vi "GV-StartPreset.vi"(8 "error in (no error)":errorcluster, 11 "Gviewer in":refnum<class "Gviewer.lvclass">) -> (0 "error out":errorcluster, 3 "Gviewer out":refnum<class "Gviewer.lvclass">)   [LabVIEW 2020, in "Sgraph_lib_V1.lvlib" / "Gviewer.lvclass"]
uses:
  Gviewer.lvclass
  Gviewer.lvclass/Gviewer.ctl
  controls/EditTagOneTag.ctl
panel:
  in  "Selector":i32[](listbox)
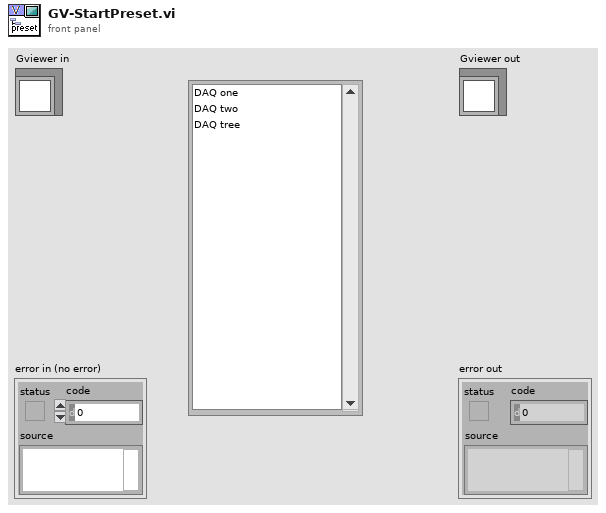
[diagram p1: front panel]
types:
  T1 = cluster{"Editor_ref":refnum<vi>, "Cnt_names":string[], "Cnt_refs":refnum<vi>[]}
  T2 = enum32{"Invalid", "Standard", "Closed", "Hidden", "Minimized", "Maximized"}
  T3 = typedef "Sgraph_lib_V1.lvlib/Gviewer.lvclass/EditTagOneTag.ctl" = cluster{"TAG":string, "min":dbl, "max":dbl, "Color":u32}
  T4 = typedef "Sgraph_lib_V1.lvlib/Gviewer.lvclass/Typedef_SelProperties.ctl" = cluster{"Color":u32, "LineType":T5, "max":dbl, "min":dbl}
  T5 = typedef "Sgraph_lib_V1.lvlib/Gviewer.lvclass/Typedef_LineType.ctl" = enum16{"num_bare", "num_MinMax_Area", "num_MinMax_Lines", "num_MinMax_Forfor", "num_Max_Area", "num_Max_Line", "num_Max_Forfor", "num_Min_Area", "num_Min_Line", "num_Min_Fosfor", "Boolean_Line_01", "Boolean_Area_01", "Boolean_Fosfor_01", "Boolean_Line_TF", "Boolean_Area_TF", "Boolean_Fosfor_TF", "Boolean_OnOff_Line", "Boolean_OnOff_Area", "Boolean_OnOff_Fosfor", "Boolean_spare", "StringEvent_Line", "StringEvent_TimeLine"}
  T6 = typedef "Sgraph_lib_V1.lvlib/DBAL_TAGprops.ctl" = T7[]
  T7 = typedef "Sgraph_lib_V1.lvlib/DBAL_TAGpropEdit.ctl" = cluster{"TAG":string, "Qtype":string, "TAGprop":T8}
  T8 = typedef "Sgraph_lib_V1.lvlib/typedef_com_TagProp.ctl" = cluster{"Description":string, "EngUnits":string, "RangeH":dbl, "RangeL":dbl, "Resolution":i32, "Obsolete":bool, "ChangeDate":timestamp, "ChangeSource":string, "ChangeReason":string, "TagFunc":u32}
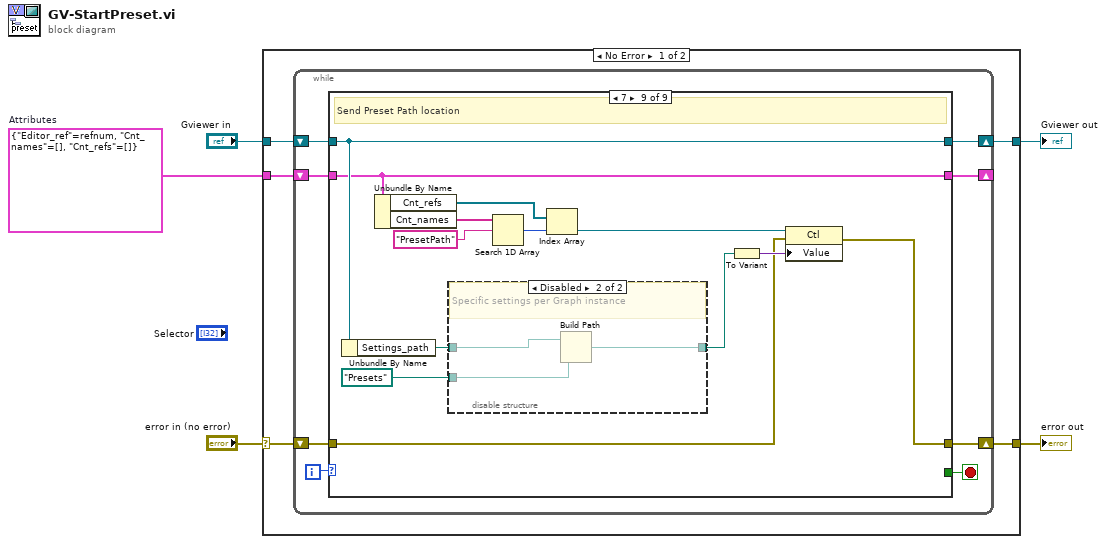
[diagram p0: block diagram]
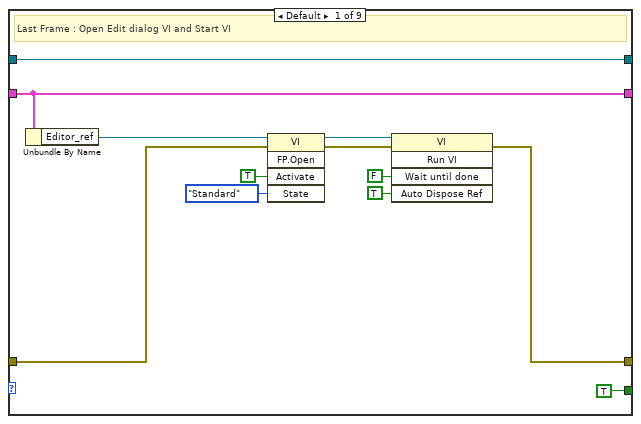
[diagram p2: hidden frame]
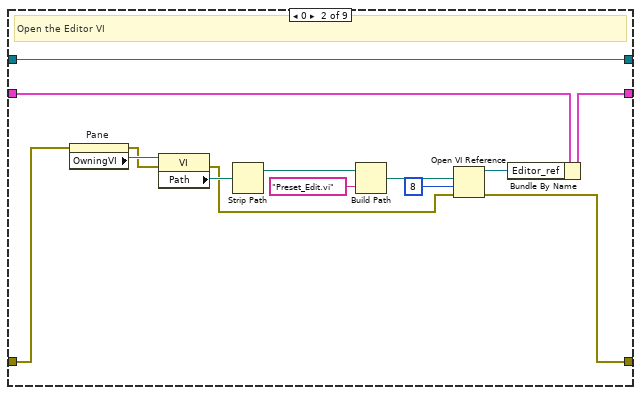
[diagram p3: hidden frame]
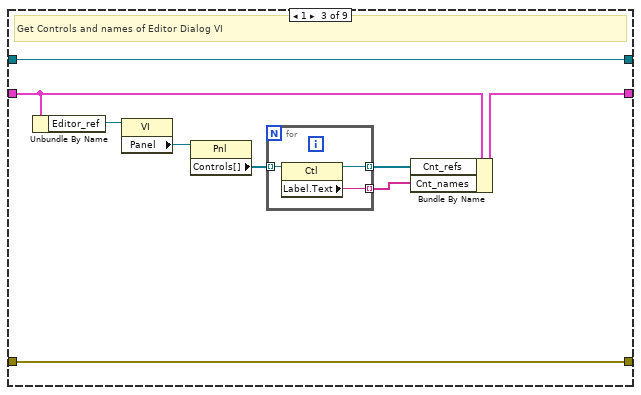
[diagram p4: hidden frame]
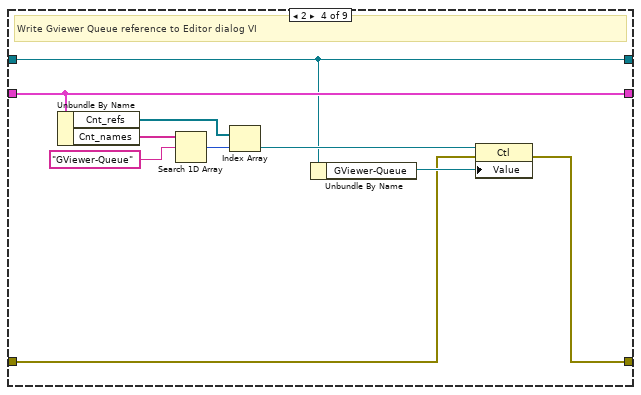
[diagram p5: hidden frame]
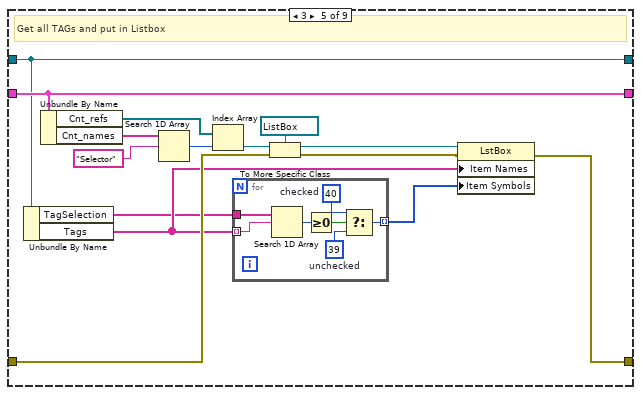
[diagram p6: hidden frame]
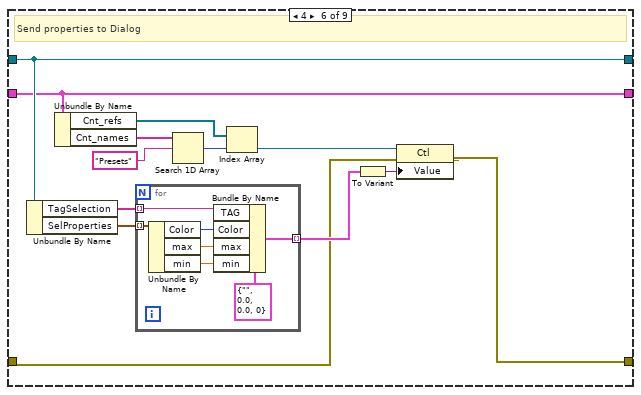
[diagram p7: hidden frame]
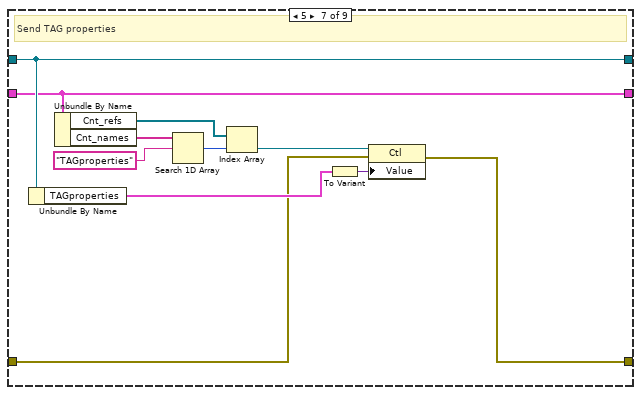
[diagram p8: hidden frame]
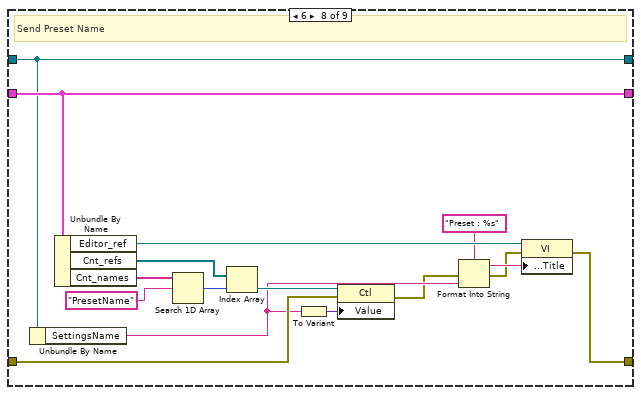
[diagram p9: hidden frame]
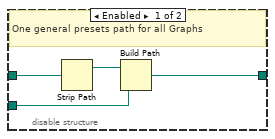
[diagram p10: hidden frame]
diagram:
  w1 = T1 {"Editor_ref"=refnum, "Cnt_names"=[], "Cnt_refs"=[]}  # Attributes
  n1 = case shown="No Error" "error in (no error)" {
    selector: "error in (no error)" -> [w9 w157]
    tunnel: [w7 w157] -> w4
    tunnel: [w8 w156] -> w2
    tunnel: "Gviewer in" -> [w10 w156]
    tunnel: w1 -> [w6 _]
    frame No Error {
      n2 = while {
        shift-right: [w15] -> w8
        shift-left: w10 -> [w17]
        shift-right: [w14] -> w7
        shift-left: w9 -> [w16]
        shift-right: [w11] -> _
        shift-left: w6 -> [w12]
        i -> [w18]
        stop <- w13 stop-if-true
        n3 = case shown="7" w18 {
          tunnel: w17 -> [w30 w44 w53 w59 w73 w101 w119 w125 w148]
          tunnel: w16 -> [w26 w31 w52 w57 w70 w89 w109 w128 w139]
          tunnel: [w30 w44 w53 w59 w73 w101 w119 w125 w148] -> w15
          tunnel: [w21 w35 w52 w58 w71 w91 w112 w126 w141] -> w14
          tunnel: [TRUE _ _ _ _ _ _ _ _] -> w13
          tunnel: [w28 w38 w46 w61 w74 w94 w114 w131 w143] -> w11
          tunnel: w12 -> [w28 w39 w45 w61 w74 w94 w114 w131 w143]
          frame Default {
            # "Last Frame : Open Edit dialog VI and Start VI"
            n4 = Unbundle By Name(w28) -> ("Editor_ref"=w25:refnum<vi>)
            n5 = invoke class="VI" method="FP.Open"(reference=w25, error in=w26, "Activate"=TRUE ("Wait Until Done"), "State"=T2."Standard") -> (reference out=w23:refnum<vi>, error out=w22:errorcluster)  [unwired: 1 in, 3 out]
            n6 = invoke class="VI" method="Run VI"(reference=w23, error in=w22, "Wait until done"=FALSE ("Wait Until Done"), "Auto Dispose Ref"=TRUE ("Auto Dispose Reference")) -> (error out=w21:errorcluster)  [unwired: 1 in, 4 out]
          }
          frame 0 {
            # "Open the Editor VI"
            n7 = property on="Pane" class="Pane"(error in=w31) -> (error out=w32:errorcluster, "OwningVI"=w33:refnum<vi>)  [unwired: 1 in, 1 out]
            n8 = property class="VI"(reference=w33, error in=w32) -> (error out=w36:errorcluster, "Path"=w43:path)  [unwired: 1 out]
            n9 = Strip Path(path=w43) -> (stripped path=w42:path)  [unwired: 1 out]
            n10 = Build Path(base path=w42, name or relative path="Preset_Edit.vi") -> (appended path=w40:path)
            n11 = Open VI Reference(vi path=w40, options=8, error in (no error)=w36) -> (vi reference=w37:refnum<vi>, error out=w35:errorcluster)  [unwired: 3 in]
            n12 = Bundle By Name(cluster=w39, "Editor_ref"=w37) -> (w38:T1)
          }
          frame 1 {
            # "Get Controls and names of Editor Dialog VI"
            n13 = Unbundle By Name(w45) -> ("Editor_ref"=w51:refnum<vi>)
            n14 = property class="VI"(reference=w51) -> ("Panel"=w50:refnum<vi>)  [unwired: 1 in, 2 out]
            n15 = property class="Pnl"(reference=w50) -> ("Controls[]"=w49:refnum<vi>[])  [unwired: 1 in, 2 out]
            n16 = for {
              tunnel: w49 -> [w56] mode=indexing
              tunnel: [w55] -> w47 mode=indexing
              tunnel: [w54] -> w48 mode=indexing
              n17 = property class="Ctl"(reference=w56) -> (reference out=w55:refnum<vi>, "Label.Text"=w54:string)  [unwired: 1 in, 1 out]
            }
            n18 = Bundle By Name(cluster=w45, "Cnt_refs"=w47, "Cnt_names"=w48) -> (w46:T1)
          }
          frame 2 {
            # "Write Gviewer Queue reference to Editor dialog VI"
            n19 = Unbundle By Name(w61) -> ("Cnt_refs"=w64:refnum<vi>[], "Cnt_names"=w66:string[])
            n20 = Search 1D Array(1D array=w66, element="GViewer-Queue") -> (index of element=w63:i32)  [unwired: 1 in]
            n21 = Index Array(array=w64, index=w63) -> (element=w62:refnum<vi>)
            n22 = Unbundle By Name(w59) -> ("GViewer-Queue"=w60:refnum<queue>)
            n23 = property class="Ctl"(reference=w62, error in=w57, "Value"=w60) -> (error out=w58:errorcluster)  [unwired: 1 out]
          }
          frame 3 {
            # "Get all TAGs and put in Listbox"
            n24 = Unbundle By Name(w73) -> ("TagSelection"=w68:string[], "Tags"=w69:string[])
            n25 = Unbundle By Name(w74) -> ("Cnt_refs"=w80:refnum<vi>[], "Cnt_names"=w81:string[])
            n26 = Search 1D Array(1D array=w81, element="Selector") -> (index of element=w79:i32)  [unwired: 1 in]
            n27 = Index Array(array=w80, index=w79) -> (element=w77:refnum<vi>)
            n28 = for {
              tunnel: w69 -> [w87] mode=indexing
              tunnel: w68 -> [w88]
              tunnel: [w82] -> w67 mode=indexing
              w83 = 40  # checked
              w84 = 39  # unchecked
              n29 = Search 1D Array(1D array=w88, element=w87) -> (index of element=w86:i32)  [unwired: 1 in]
              n30 = Greater Or Equal To 0?(x=w86) -> (x >= 0?=w85:bool)
              n31 = Select(t=w83, s=w85, f=w84) -> (s? t:f=w82:i32)
            }
            n32 = To More Specific Class(target class=refnum<vi> refnum ("Selector"), reference=w77, error in=w70) -> (specific class reference=w75:refnum<vi>, error out=w72:errorcluster)
            n33 = property class="LstBox"(reference=w75, error in=w72, "Item Names"=w69, "Item Symbols"=w67) -> (error out=w71:errorcluster)  [unwired: 1 out]
          }
          frame 4 {
            # "Send properties to Dialog"
            n34 = Unbundle By Name(w101) -> ("TagSelection"=w100:string[], "SelProperties"=w99:T4[])
            n35 = Unbundle By Name(w94) -> ("Cnt_refs"=w97:refnum<vi>[], "Cnt_names"=w98:string[])
            n36 = for {
              tunnel: w100 -> [w106] mode=indexing
              tunnel: w99 -> [w108] mode=indexing
              tunnel: [w102] -> w93 mode=indexing
              n37 = Unbundle By Name(w108) -> ("Color"=w105:u32, "max"=w104:dbl, "min"=w103:dbl)
              n38 = Bundle By Name(cluster=T3 {"TAG"="", "min"=0.0, "max"=0.0, "Color"=0} ("Selected-Tag"), "TAG"=w106, "Color"=w105, "max"=w104, "min"=w103) -> (w102:T3)
            }
            n39 = Search 1D Array(1D array=w98, element="Presets") -> (index of element=w96:i32)  [unwired: 1 in]
            n40 = Index Array(array=w97, index=w96) -> (element=w90:refnum<vi>)
            n41 = To Variant(anything=w93) -> (Variant=w92:variant)
            n42 = property class="Ctl"(reference=w90, error in=w89, "Value"=w92) -> (error out=w91:errorcluster)  [unwired: 1 out]
          }
          frame 5 {
            # "Send TAG properties"
            n43 = Unbundle By Name(w119) -> ("TAGproperties"=w111:T6)
            n44 = Unbundle By Name(w114) -> ("Cnt_refs"=w117:refnum<vi>[], "Cnt_names"=w118:string[])
            n45 = Search 1D Array(1D array=w118, element="TAGproperties") -> (index of element=w116:i32)  [unwired: 1 in]
            n46 = Index Array(array=w117, index=w116) -> (element=w110:refnum<vi>)
            n47 = To Variant(anything=w111) -> (Variant=w113:variant)
            n48 = property class="Ctl"(reference=w110, error in=w109, "Value"=w113) -> (error out=w112:errorcluster)  [unwired: 1 out]
          }
          frame 6 {
            # "Send Preset Name"
            n49 = Unbundle By Name(w125) -> ("SettingsName"=w123:string)
            n50 = Unbundle By Name(w131) -> ("Editor_ref"=w127:refnum<vi>, "Cnt_refs"=w134:refnum<vi>[], "Cnt_names"=w135:string[])
            n51 = Search 1D Array(1D array=w135, element="PresetName") -> (index of element=w133:i32)  [unwired: 1 in]
            n52 = Index Array(array=w134, index=w133) -> (element=w129:refnum<vi>)
            n53 = To Variant(anything=w123) -> (Variant=w130:variant)
            n54 = property class="Ctl"(reference=w129, error in=w128, "Value"=w130) -> (error out=w121:errorcluster)  [unwired: 1 out]
            n55 = Format Into String(format string="Preset : %s", error in=w121, w123) -> (resulting string=w122:string, error out=w120:errorcluster)  [unwired: 1 in]
            n56 = property class="VI"(reference=w127, error in=w120, "Front Panel.Title"=w122) -> (error out=w126:errorcluster)  [unwired: 1 out]
          }
          frame 7 {
            # "Send Preset Path location"
            n57 = Unbundle By Name(w148) -> ("Settings_path"=w138:path)
            n58 = Unbundle By Name(w143) -> ("Cnt_refs"=w146:refnum<vi>[], "Cnt_names"=w147:string[])
            n59 = disable-structure shown="Disabled" {
              disable-tunnel: w138 -> [w152 w153]
              disable-tunnel: path "Presets" ("name or relative path") -> [w150 w155]
              disable-tunnel: [w149 w154] -> w136
              frame Enabled {
                # "One general presets path for all Graphs"
                n60 = Strip Path(path=w152) -> (stripped path=w151:path)  [unwired: 1 out]
                n61 = Build Path(base path=w151, name or relative path=w150) -> (appended path=w149:path)
              }
              frame Disabled {
                # "Specific settings per Graph instance"
                n62 = Build Path(base path=w153, name or relative path=w155) -> (appended path=w154:path)
              }
            }
            n63 = Search 1D Array(1D array=w147, element="PresetPath") -> (index of element=w145:i32)  [unwired: 1 in]
            n64 = Index Array(array=w146, index=w145) -> (element=w140:refnum<vi>)
            n65 = To Variant(anything=w136) -> (Variant=w142:variant)
            n66 = property class="Ctl"(reference=w140, error in=w139, "Value"=w142) -> (error out=w141:errorcluster)  [unwired: 1 out]
          }
        }
      }
    }
    frame Error {
    }
  }
  "error out" <- w4
  "Gviewer out" <- w2
